vi "Get World extent.vi"(0 "Triangles":T1[](array[typedef])) -> (1 "Pmax (x, y, z)":sgl[](array[numeric]), 2 "Pmin (x, y, z)":sgl[](array[numeric]))   [LabVIEW 2014]
uses:
  Typedefs/Triangle.ctl
panel:
  # "PN 18/01/2015"
  # "Vertices"
  # "Edges"
  # "Unit normal"
  # "pre-store"
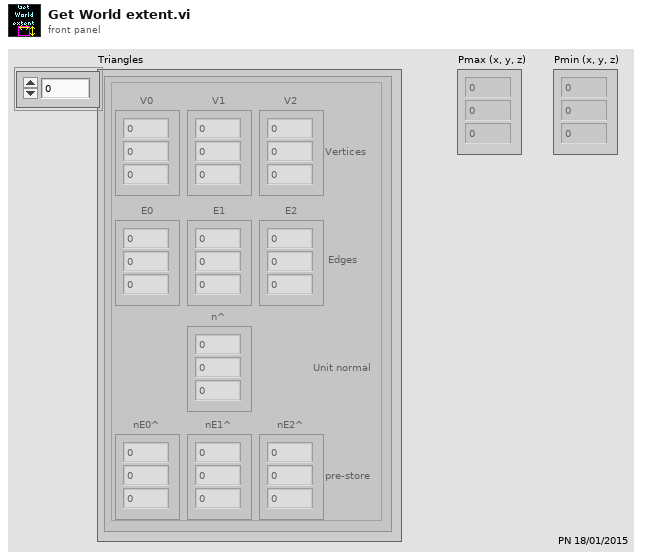
[diagram p1: front panel]
types:
  T1 = typedef "Triangle.ctl" = cluster{"V0":sgl[], "V1":sgl[], "V2":sgl[], "E0":sgl[], "E1":sgl[], "E2":sgl[], "n^":sgl[], "nE0^":sgl[], "nE1^":sgl[], "nE2^":sgl[]}
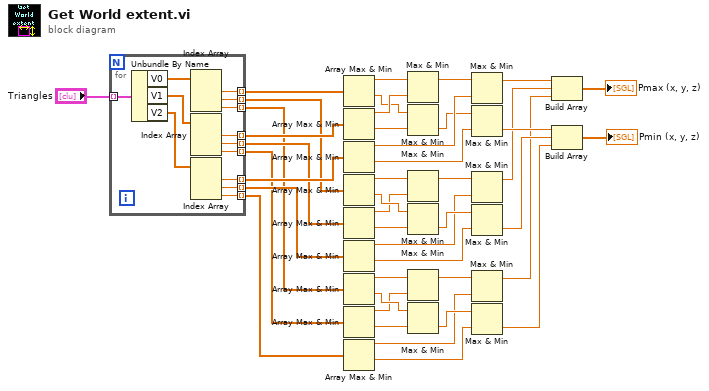
[diagram p0: block diagram]
diagram:
  n1 = for {
    tunnel: "Triangles" -> [w55] mode=indexing
    tunnel: [w51] -> w41 mode=indexing
    tunnel: [w50] -> w36 mode=indexing
    tunnel: [w49] -> w33 mode=indexing
    tunnel: [w48] -> w38 mode=indexing
    tunnel: [w47] -> w35 mode=indexing
    tunnel: [w46] -> w32 mode=indexing
    tunnel: [w45] -> w37 mode=indexing
    tunnel: [w44] -> w34 mode=indexing
    tunnel: [w43] -> w31 mode=indexing
    n2 = Unbundle By Name(w55) -> ("V0"=w54:sgl[], "V1"=w53:sgl[], "V2"=w52:sgl[])
    n3 = Index Array(array=w54) -> (element #1=w51:sgl, element #2=w50:sgl, element #3=w49:sgl)  [unwired: 3 in]
    n4 = Index Array(array=w53) -> (element #1=w48:sgl, element #2=w47:sgl, element #3=w46:sgl)  [unwired: 3 in]
    n5 = Index Array(array=w52) -> (element #1=w45:sgl, element #2=w44:sgl, element #3=w43:sgl)  [unwired: 3 in]
  }
  n6 = Array Max & Min(array=w41) -> (max value=w30:sgl, min value=w25:sgl)  [unwired: 2 out]
  n7 = Array Max & Min(array=w38) -> (max value=w29:sgl, min value=w24:sgl)  [unwired: 2 out]
  n8 = Array Max & Min(array=w37) -> (max value=w27:sgl, min value=w22:sgl)  [unwired: 2 out]
  n9 = Array Max & Min(array=w36) -> (max value=w18:sgl, min value=w17:sgl)  [unwired: 2 out]
  n10 = Array Max & Min(array=w35) -> (max value=w16:sgl, min value=w15:sgl)  [unwired: 2 out]
  n11 = Array Max & Min(array=w34) -> (max value=w14:sgl, min value=w13:sgl)  [unwired: 2 out]
  n12 = Array Max & Min(array=w33) -> (max value=w8:sgl, min value=w7:sgl)  [unwired: 2 out]
  n13 = Array Max & Min(array=w32) -> (max value=w6:sgl, min value=w5:sgl)  [unwired: 2 out]
  n14 = Array Max & Min(array=w31) -> (max value=w4:sgl, min value=w3:sgl)  [unwired: 2 out]
  n15 = Max & Min(x=w30, y=w29) -> (max(x,y)=w28:sgl)  [unwired: 1 out]
  n16 = Max & Min(x=w25, y=w24) -> (min(x,y)=w23:sgl)  [unwired: 1 out]
  n17 = Max & Min(x=w18, y=w16) -> (max(x,y)=w19:sgl)  [unwired: 1 out]
  n18 = Max & Min(x=w17, y=w15) -> (min(x,y)=w20:sgl)  [unwired: 1 out]
  n19 = Max & Min(x=w8, y=w6) -> (max(x,y)=w10:sgl)  [unwired: 1 out]
  n20 = Max & Min(x=w7, y=w5) -> (min(x,y)=w9:sgl)  [unwired: 1 out]
  n21 = Max & Min(x=w28, y=w27) -> (max(x,y)=w26:sgl)  [unwired: 1 out]
  n22 = Max & Min(x=w23, y=w22) -> (min(x,y)=w21:sgl)  [unwired: 1 out]
  n23 = Max & Min(x=w19, y=w14) -> (max(x,y)=w12:sgl)  [unwired: 1 out]
  n24 = Max & Min(x=w20, y=w13) -> (min(x,y)=w11:sgl)  [unwired: 1 out]
  n25 = Max & Min(x=w10, y=w4) -> (max(x,y)=w2:sgl)  [unwired: 1 out]
  n26 = Max & Min(x=w9, y=w3) -> (min(x,y)=w1:sgl)  [unwired: 1 out]
  n27 = Build Array(w26, w12, w2) -> (→"Pmax (x, y, z)":sgl[])
  n28 = Build Array(w21, w11, w1) -> (→"Pmin (x, y, z)":sgl[])
